vi "_Convert to DAC Value.vi"(4 "Type":u8, 6 "Neg Polarity (F)":bool, 8 "Offset":dbl, 9 "Slop":dbl, 10 "Number":dbl, 11 "Channel":i32=1) -> (1 "DAC Value":i32)   [LabVIEW 2015]
uses:
  _Global Configuration.vi
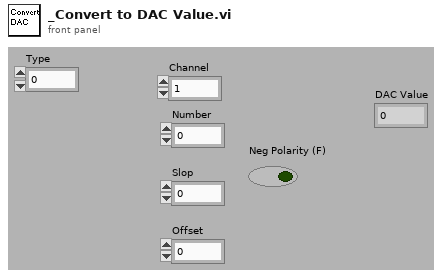
[diagram p1: front panel]
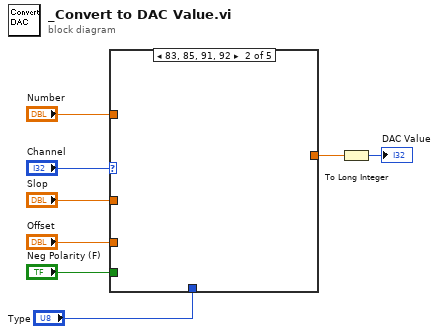
[diagram p0: block diagram]
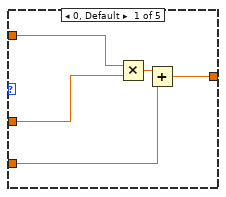
[diagram p2: hidden frame]
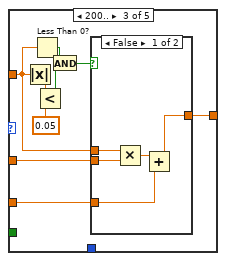
[diagram p3: hidden frame]
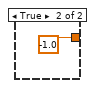
[diagram p4: hidden frame]
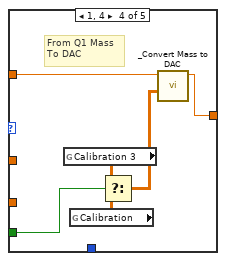
[diagram p5: hidden frame]
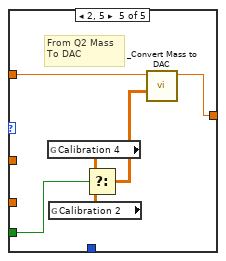
[diagram p6: hidden frame]
diagram:
  n1 = case shown="83, 85, 91, 92" "Channel" {
    tunnel: "Number" -> [w13 _ w15 w34 w40]
    tunnel: [w12 _ w17 w33 w39] -> w6
    tunnel: "Slop" -> [w10 _ w16 _ _]
    tunnel: "Offset" -> [w9 _ w14 _ _]
    tunnel: "Neg Polarity (F)" -> [_ _ _ w30 w38]
    tunnel: "Type" -> [_ _ _ _ _]
    frame 0, Default {
      n2 = Multiply(x=w13, y=w10) -> (x*y=w11:dbl)
      n3 = Add(x=w11, y=w9) -> (x+y=w12:dbl)
    }
    frame 83, 85, 91, 92 {
    }
    frame 200.. {
      n4 = Absolute Value(x=w15) -> (abs(x)=w21:dbl)
      n5 = Less Than 0?(x=w15) -> (x < 0?=w19:bool)
      n6 = Less?(x=w21, y=0.05) -> (x < y?=w18:bool)
      n7 = And(x=w19, y=w18) -> (x .and. y?=w20:bool)
      n8 = case shown="False" w20 {
        tunnel: [w23 -1.0 ("y")] -> w17
        tunnel: w16 -> [w26 _]
        tunnel: w15 -> [w25 _]
        tunnel: w14 -> [w24 _]
        frame False {
          n9 = Multiply(x=w25, y=w26) -> (x*y=w27:dbl)
          n10 = Add(x=w27, y=w24) -> (x+y=w23:dbl)
        }
        frame True {
        }
      }
    }
    frame 1, 4 {
      # "From Q1 Mass\nTo DAC"
      n11 = global read "_Global Configuration.vi" "Calibration 3"() -> (w32:dbl[][])
      n12 = global read "_Global Configuration.vi" "Calibration"() -> (w31:dbl[][])
      n13 = Select(t=w32, s=w30, f=w31) -> (s? t:f=w29:dbl[][])
      n14 = call "_Convert Mass to DAC.vi"("Calibration Table"=w29, "Mass"=w34) -> ("DAC Value"=w33:dbl)  [unwired: 2 in, 3 out]
    }
    frame 2, 5 {
      # "From Q2 Mass\nTo DAC"
      n15 = global read "_Global Configuration.vi" "Calibration 4"() -> (w37:dbl[][])
      n16 = global read "_Global Configuration.vi" "Calibration 2"() -> (w36:dbl[][])
      n17 = Select(t=w37, s=w38, f=w36) -> (s? t:f=w35:dbl[][])
      n18 = call "_Convert Mass to DAC.vi"("Calibration Table"=w35, "Mass"=w40) -> ("DAC Value"=w39:dbl)  [unwired: 2 in, 3 out]
    }
  }
  n19 = To Long Integer(number=w6) -> (32bit integer=→"DAC Value":i32)
